vi "ABB Delete Report field.vi"(7 "Delete":bool, 9 "End":string, 10 "Start":string, 11 "Report in":string) -> (3 "Report out":string)   [LabVIEW 2017]
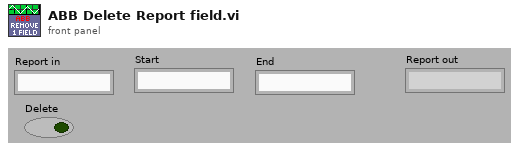
[diagram p1: front panel]
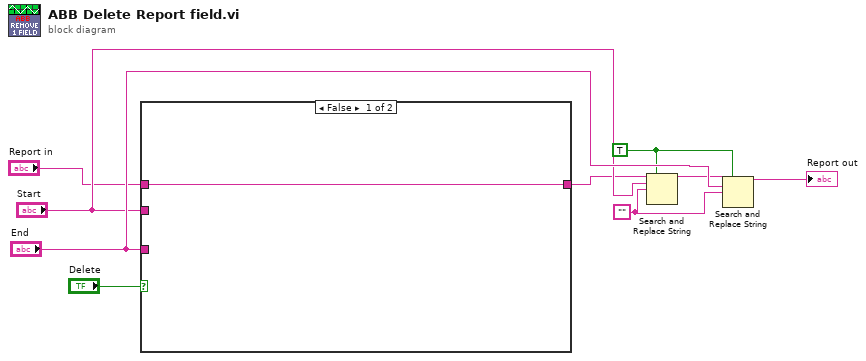
[diagram p0: block diagram]
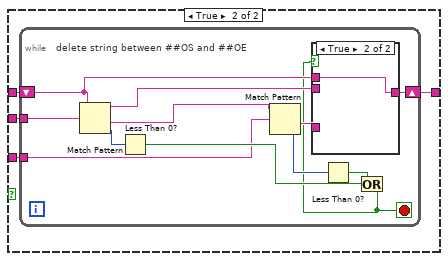
[diagram p2: hidden frame]
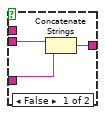
[diagram p3: hidden frame]
diagram:
  w2 = TRUE ("replace all? (F)")
  w3 = "" ("replace string (\"\")")
  n1 = case shown="False" "Delete" {
    tunnel: "End" -> [_ w14]
    tunnel: "Start" -> [_ w13]
    tunnel: [w10 w12] -> w7
    tunnel: "Report in" -> [w10 w11]
    frame False {
    }
    frame True {
      n2 = while {
        shift-right: [w24] -> w12
        shift-left: w11 -> [w18]
        tunnel: w13 -> [w16]
        tunnel: w14 -> [w15]
        stop <- w17 stop-if-true
        # "delete string between ##OS and ##OE"
        n3 = Match Pattern(string=w18, regular expression=w16) -> (before substring=w25:string, after substring=w19:string, offset past match=w26:i32)  [unwired: 1 in, 1 out]
        n4 = Less Than 0?(x=w26) -> (x < 0?=w20:bool)
        n5 = Match Pattern(string=w19, regular expression=w15) -> (after substring=w23:string, offset past match=w22:i32)  [unwired: 1 in, 2 out]
        n6 = Less Than 0?(x=w22) -> (x < 0?=w21:bool)
        n7 = Or(x=w21, y=w20) -> (x .or. y?=w17:bool)
        n8 = case shown="True" w17 {
          tunnel: w25 -> [w29 _]
          tunnel: [w28 w30] -> w24
          tunnel: w23 -> [w27 _]
          tunnel: w18 -> [_ w30]
          frame False {
            n9 = Concatenate Strings(w29, w27) -> (w28:string)
          }
          frame True {
          }
        }
      }
    }
  }
  n10 = Search and Replace String(replace all?=w2, input string=w7, search string="Start", replace string=w3) -> (result string=w4:string)  [unwired: 4 in, 3 out]
  n11 = Search and Replace String(replace all?=w2, input string=w4, search string="End", replace string=w3) -> (result string=→"Report out":string)  [unwired: 4 in, 3 out]
